vi "Example.vi"() -> ()   [LabVIEW 2013]
uses:
  Message que instance modes enum.ctl
  Example msgQ names enums.ctl
  Interloop MessageQ.lvlib
panel:
  out "Message C":string
  out "Message B":string
  in  "stop":bool
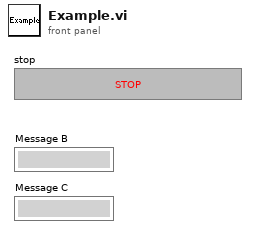
[diagram p1: front panel]
types:
  T1 = typedef "Interloop MessageQ.lvlib/Message que instance modes enum.ctl" = enum16{"Initialize", "Broadcast Message", "Send Message", "Read Message", "Kill"}
  T2 = typedef "Example msgQ names enums.ctl" = enum16{"Loop A", "Loop B", "Loop C"}
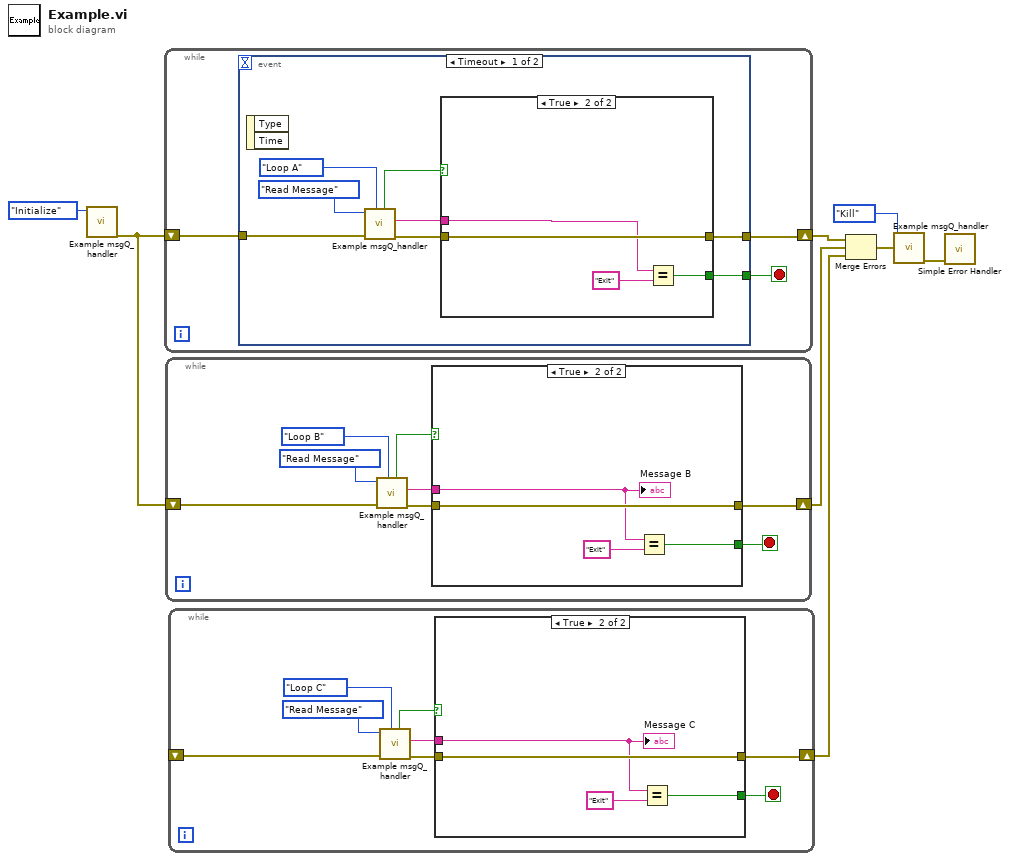
[diagram p0: block diagram]
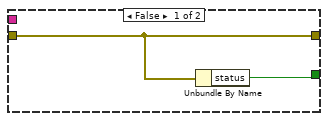
[diagram p2: hidden frame]
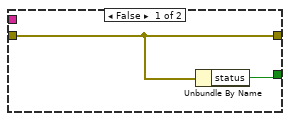
[diagram p3: hidden frame]
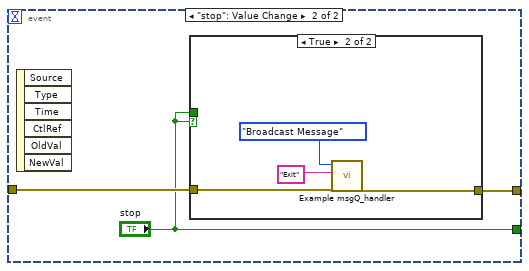
[diagram p4: hidden frame]
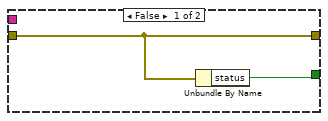
[diagram p6: hidden frame]
diagram:
  n1 = call "Example msgQ_handler.vi"("Mode"=Message_que_instance_modes_enum."Initialize") -> ("error out"=w3:errorcluster)  [unwired: 4 in, 6 out]
  n2 = while {
    shift-right: [w10] -> w2
    shift-left: w3 -> [w11]
    stop <- w9 stop-if-true
    n3 = event shown="[0] Timeout" {
      selector: _ -> [_ _]
      dyn-events: _ -> [_ _]
      timeout: _ -> [_ _]
      tunnel: w11 -> [w19 w28]
      tunnel: [w14 w27] -> w10
      tunnel: [w13 "stop"] -> w9
      event Timeout {
        n4 = event-data() -> ()  [unwired: 3 out]
        n5 = call "Example msgQ_handler.vi"("MsgQ enum"=Example_msgQ_names_enums."Loop A", "error in (no error)"=w19, "Mode"=Message_que_instance_modes_enum."Read Message") -> ("error out"=w16:errorcluster, "Message Received String"=w15:string, "Message Recieved?"=w12:bool)  [unwired: 2 in, 4 out]
        n6 = case shown="True" w12 {
          tunnel: w16 -> [w20 w25]
          tunnel: w15 -> [_ w22]
          tunnel: [w20 w25] -> w14
          tunnel: [w21 w23] -> w13
          frame False {
            n7 = Unbundle By Name(w20) -> ("status"=w21:bool)
          }
          frame True {
            n8 = Equal?(x=w22, y="Exit") -> (x = y?=w23:bool)
          }
        }
      }
      event "stop": Value Change {
        n9 = event-data() -> ()  [unwired: 7 out]
        n10 = case shown="True" "stop" {
          tunnel: w28 -> [w29 w33]
          tunnel: "stop" -> [_ _]
          tunnel: [w29 w31] -> w27
          frame False {
          }
          frame True {
            n11 = call "Example msgQ_handler.vi"("error in (no error)"=w33, "Message Send String"="Exit" ("Message String"), "Mode"=Message_que_instance_modes_enum."Broadcast Message") -> ("error out"=w31:errorcluster)  [unwired: 2 in, 6 out]
          }
        }
      }
    }
  }
  n12 = while {
    shift-right: [w36] -> w4
    shift-left: w3 -> [w41]
    stop <- w35 stop-if-true
    n13 = call "Example msgQ_handler.vi"("MsgQ enum"=Example_msgQ_names_enums."Loop B", "error in (no error)"=w41, "Mode"=Message_que_instance_modes_enum."Read Message") -> ("error out"=w38:errorcluster, "Message Received String"=w37:string, "Message Recieved?"=w34:bool)  [unwired: 2 in, 4 out]
    n14 = case shown="True" w34 {
      tunnel: w38 -> [w42 w47]
      tunnel: w37 -> [_ w44]
      tunnel: [w42 w47] -> w36
      tunnel: [w43 w45] -> w35
      frame False {
        n15 = Unbundle By Name(w42) -> ("status"=w43:bool)
      }
      frame True {
        n16 = Equal?(x=w44, y="Exit") -> (x = y?=w45:bool)
        "Message B" <- w44
      }
    }
  }
  n17 = while {
    shift-right: [w50] -> w1
    shift-left: _ -> [w55]
    stop <- w49 stop-if-true
    n18 = call "Example msgQ_handler.vi"("MsgQ enum"=Example_msgQ_names_enums."Loop C", "error in (no error)"=w55, "Mode"=Message_que_instance_modes_enum."Read Message") -> ("error out"=w52:errorcluster, "Message Received String"=w51:string, "Message Recieved?"=w48:bool)  [unwired: 2 in, 4 out]
    n19 = case shown="True" w48 {
      tunnel: w52 -> [w56 w61]
      tunnel: w51 -> [_ w58]
      tunnel: [w56 w61] -> w50
      tunnel: [w57 w59] -> w49
      frame False {
        n20 = Unbundle By Name(w56) -> ("status"=w57:bool)
      }
      frame True {
        n21 = Equal?(x=w58, y="Exit") -> (x = y?=w59:bool)
        "Message C" <- w58
      }
    }
  }
  n22 = Merge Errors(w2, w4, w1) -> (w7:errorcluster)
  n23 = call "Example msgQ_handler.vi"("error in (no error)"=w7, "Mode"=Message_que_instance_modes_enum."Kill") -> ("error out"=w6:errorcluster)  [unwired: 3 in, 6 out]
  n24 = call <vilib>:"Simple Error Handler.vi"("error in (no error)"=w6) -> ()  [unwired: 1 in, 8 out]
